vi "3kButtons2D22x22.vi"() -> ()   [LabVIEW 2011]
doc: "3000 buttons from haobo.li@pansino.com.cn\nhttp://www.linkedin.com/pub/haobo-li/17/8a/220\nthanks to\nhttp://www.fatcow.com/free-icons"
panel:
  out "zoom":bool
  out "youtube":bool
  out "yelp":bool
  out "yellow_submarine":bool
  out "yahoo_messenger":bool
  out "yacht":bool
  out "xing":bool
  out "xhtml_valid":bool
  out "xhtml_go":bool
  out "xhtml_delete":bool
  out "xhtml_add":bool
  out "xhtml":bool
  out "x_ray":bool
  out "www_page":bool
  out "wrench_orange":bool
  out "wrench":bool
  out "wrapping_tight":bool
  out "wrapping_square":bool
  out "wrapping_magazine":bool
  out "wrapping_inline":bool
  out "wrapping_in_front":bool
  out "wrapping_edit":bool
  out "wrapping_between":bool
  out "wrapping_behind":bool
  out "world_link":bool
  out "world_go":bool
  out "world_edit":bool
  out "world_delete":bool
  out "world_add":bool
  out "world":bool
  out "workspace":bool
  out "wordpress_blog":bool
  out "wordpress":bool
  out "wizard_women":bool
  out "wizard":bool
  out "wishlist_add":bool
  out "winrar_view":bool
  out "winrar_extract":bool
  out "winrar_add":bool
  out "wine_pairings":bool
  out "windy":bool
  out "widgets":bool
  out "widescreen":bool
  out "whistle":bool
  out "weight":bool
  out "weighing_mashine":bool
  out "webcam_error":bool
  out "webcam_delete":bool
  out "webcam_add":bool
  out "webcam":bool
  out "web_concierge":bool
  out "weather_sun":bool
  out "weather_snow":bool
  out "weather_rain":bool
  out "weather_lightning":bool
  out "weather_cloudy":bool
  out "weather_clouds":bool
  out "wand":bool
  out "wallet":bool
  out "walk":bool
  out "vslider":bool
  out "vrule":bool
  out "vlc":bool
  out "visa_electron":bool
  out "visa_2":bool
  out "visa":bool
  out "virus_protection":bool
  out "virb":bool
  out "vimeo":bool
  out "viewstack":bool
  out "videodisplay":bool
  out "video_mode":bool
  out "video":bool
  out "viddler":bool
  out "vhs":bool
  out "vector_delete":bool
  out "vector_add":bool
  out "vector":bool
  out "vdividedbox":bool
  out "vcard_edit":bool
  out "vcard_delete":bool
  out "vcard_add":bool
  out "vcard":bool
  out "vbox":bool
  out "user_zorro":bool
  out "user_yoda":bool
  out "user_wicket":bool
  out "user_waiter_female_black":bool
  out "user_waiter_female":bool
  out "user_waiter":bool
  out "user_viking_female":bool
  out "user_viking":bool
  out "user_vietnamese_female":bool
  out "user_vietnamese":bool
  out "user_trooper_captain":bool
  out "user_trooper":bool
  out "user_swimmer_female":bool
  out "user_swimmer_black":bool
  out "user_swimmer":bool
  out "user_superman":bool
  out "user_suit":bool
  out "user_student_female_black":bool
  out "user_student_female":bool
  out "user_student_black":bool
  out "user_student":bool
  out "user_striper_black":bool
  out "user_striper":bool
  out "user_stewardess_black":bool
  out "user_stewardess":bool
  out "user_squidward":bool
  out "user_sponge_bob":bool
  out "user_spiderman":bool
  out "user_soldier":bool
  out "user_silhouette":bool
  out "user_scream":bool
  out "user_samurai":bool
  out "user_sailor_black":bool
  out "user_sailor":bool
  out "user_robocop":bool
  out "user_redskin":bool
  out "user_red":bool
  out "user_rambo":bool
  out "user_racer":bool
  out "user_r2d2":bool
  out "user_queen_black":bool
  out "user_queen":bool
  out "user_pumpkin":bool
  out "user_priest_black":bool
  out "user_priest":bool
  out "user_policeman_black":bool
  out "user_policeman":bool
  out "user_police_female_black":bool
  out "user_police_female":bool
  out "user_police_england":bool
  out "user_plankton":bool
  out "user_pirate":bool
  out "user_pilot_civil":bool
  out "user_pilot":bool
  out "user_patrick":bool
  out "user_orange":bool
  out "user_oldwoman_black":bool
  out "user_oldwoman":bool
  out "user_oldman_black":bool
  out "user_oldman":bool
  out "user_officer_black":bool
  out "user_officer":bool
  out "user_nun_black":bool
  out "user_nun":bool
  out "user_nude_female_black":bool
  out "user_nude_female":bool
  out "user_nude_black":bool
  out "user_nude":bool
  out "user_ninja":bool
  out "user_muslim_female":bool
  out "user_muslim":bool
  out "user_mexican":bool
  out "user_medical_female_black":bool
  out "user_medical_female":bool
  out "user_medical_black":bool
  out "user_medical":bool
  out "user_maid":bool
  out "user_lisa":bool
  out "user_leprechaun":bool
  out "user_knight":bool
  out "user_king_black":bool
  out "user_king":bool
  out "user_judge_black":bool
  out "user_judge":bool
  out "user_jew":bool
  out "user_jester":bool
  out "user_jawa":bool
  out "user_jason":bool
  out "user_ironman":bool
  out "user_indian_female":bool
  out "user_indian":bool
  out "user_imprisoned_female_black":bool
  out "user_imprisoned_female":bool
  out "user_imprisoned_black":bool
  out "user_imprisoned":bool
  out "user_hendrix":bool
  out "user_halk":bool
  out "user_green":bool
  out "user_gray":bool
  out "user_goth":bool
  out "user_gomer":bool
  out "user_go":bool
  out "user_gladiator":bool
  out "user_geisha":bool
  out "user_freddy":bool
  out "user_firefighter_black":bool
  out "user_firefighter":bool
  out "user_female":bool
  out "user_eskimo_female":bool
  out "user_eskimo":bool
  out "user_emo":bool
  out "user_egyptian_female":bool
  out "user_egyptian":bool
  out "user_edit":bool
  out "user_dracula":bool
  out "user_diver":bool
  out "user_devil":bool
  out "user_detective_gray":bool
  out "user_detective":bool
  out "user_delete":bool
  out "user_death":bool
  out "user_darth_vader":bool
  out "user_crabs":bool
  out "user_cowboy_female":bool
  out "user_cowboy":bool
  out "user_cook_female_black":bool
  out "user_cook_female":bool
  out "user_cook_black":bool
  out "user_cook":bool
  out "user_comment":bool
  out "user_clown":bool
  out "user_chief_female_black":bool
  out "user_chief_female":bool
  out "user_chief_black":bool
  out "user_chief":bool
  out "user_catwomen":bool
  out "user_c3po":bool
  out "user_buddhist":bool
  out "user_boxer_black":bool
  out "user_boxer":bool
  out "user_blondy":bool
  out "user_bishop":bool
  out "user_bender":bool
  out "user_beach_lifeguard_female":bool
  out "user_beach_lifeguard":bool
  out "user_batman":bool
  out "user_bart":bool
  out "user_banker":bool
  out "user_ballplayer_black":bool
  out "user_ballplayer":bool
  out "user_astronaut":bool
  out "user_angel_female_black":bool
  out "user_angel_female":bool
  out "user_angel_black":bool
  out "user_angel":bool
  out "user_alien":bool
  out "user_add":bool
  out "user":bool
  out "usb_3":bool
  out "update":bool
  out "universal_binary":bool
  out "unicorn":bool
  out "understanding":bool
  out "underle_dictionary":bool
  out "umbrella":bool
  out "ufo":bool
  out "ubuntu":bool
  out "twitter_2":bool
  out "twitter_1":bool
  out "tux":bool
  out "turntable":bool
  out "tumblr":bool
  out "tubes":bool
  out "tub":bool
  out "trolley":bool
  out "trojan_horse":bool
  out "tree":bool
  out "travel":bool
  out "transmit_go":bool
  out "transmit_error":bool
  out "transmit_edit":bool
  out "transmit_delete":bool
  out "transmit_blue":bool
  out "transmit_add":bool
  out "transmit":bool
  out "transform_shear":bool
  out "transform_selection":bool
  out "transform_scale":bool
  out "transform_rotate_270":bool
  out "transform_rotate_180":bool
  out "transform_rotate_90":bool
  out "transform_rotate":bool
  out "transform_perspective":bool
  out "transform_path":bool
  out "transform_move":bool
  out "transform_layer":bool
  out "transform_flip":bool
  out "transform_crop_resize":bool
  out "transform_crop":bool
  out "traffic_usage":bool
  out "traffic_lights_yellow":bool
  out "traffic_lights_red":bool
  out "traffic_lights_green":bool
  out "traffic_lights":bool
  out "trade":bool
  out "tractor":bool
  out "toxic":bool
  out "tower":bool
  out "toucan":bool
  out "total_plan_cost":bool
  out "toster":bool
  out "tornado":bool
  out "torchere":bool
  out "tooth":bool
  out "toolbox":bool
  out "to_do_list_cheked_all":bool
  out "to_do_list_cheked_1":bool
  out "to_do_list":bool
  out "title_window":bool
  out "tire":bool
  out "tipper":bool
  out "timeline_marker":bool
  out "timeline":bool
  out "time_go":bool
  out "time_delete":bool
  out "time_add":bool
  out "time":bool
  out "tilelist":bool
  out "tick":bool
  out "thumb_up":bool
  out "thumb_down":bool
  out "three_tags":bool
  out "things_digital":bool
  out "things_beauty":bool
  out "theater":bool
  out "textfield_rename":bool
  out "textfield_key":bool
  out "textfield_delete":bool
  out "textfield_add":bool
  out "textfield":bool
  out "text_width":bool
  out "text_uppercase":bool
  out "text_underline":bool
  out "text_superscript":bool
  out "text_subscript":bool
  out "text_strikethroungh":bool
  out "text_smallcaps":bool
  out "text_signature":bool
  out "text_resize":bool
  out "text_replace":bool
  out "text_prose":bool
  out "text_pagination_100":bool
  out "text_pagination":bool
  out "text_padding_top":bool
  out "text_padding_right":bool
  out "text_padding_left":bool
  out "text_padding_bottom":bool
  out "text_lowercase":bool
  out "text_list_numbers":bool
  out "text_list_bullets":bool
  out "text_linespacing":bool
  out "text_letterspacing":bool
  out "text_letter_omega":bool
  out "text_large_cap":bool
  out "text_language":bool
  out "text_kerning":bool
  out "text_italic":bool
  out "text_indent_remove":bool
  out "text_indent":bool
  out "text_horizontalrule":bool
  out "text_heading_6":bool
  out "text_heading_5":bool
  out "text_heading_4":bool
  out "text_heading_3":bool
  out "text_heading_2":bool
  out "text_heading_1":bool
  out "text_dropcaps":bool
  out "text_drama":bool
  out "text_document_wrap":bool
  out "text_document":bool
  out "text_columns":bool
  out "text_bold":bool
  out "text_area":bool
  out "text_allcaps":bool
  out "text_align_right":bool
  out "text_align_left":bool
  out "text_align_justity":bool
  out "text_align_center":bool
  out "text":bool
  out "terminal_seats_red":bool
  out "terminal_seats_blue":bool
  out "terminal":bool
  out "temperature_5":bool
  out "temperature_4":bool
  out "temperature_3":bool
  out "temperature_2":bool
  out "temperature_1":bool
  out "television_delete":bool
  out "television_add":bool
  out "television":bool
  out "telephone_link":bool
  out "telephone_key":bool
  out "telephone_go":bool
  out "telephone_error":bool
  out "telephone_edit":bool
  out "telephone_delete":bool
  out "telephone_add":bool
  out "telephone":bool
  out "teddy_bear":bool
  out "technorati":bool
  out "teapot":bool
  out "tea_cup":bool
  out "tags_cloud":bool
  out "tag_yellow":bool
  out "tag_red":bool
  out "tag_purple":bool
  out "tag_pink":bool
  out "tag_orange":bool
  out "tag_green":bool
  out "tag_blue_edit":bool
  out "tag_blue_delete":bool
  out "tag_blue_add":bool
  out "tag_blue":bool
  out "tag":bool
  out "tabnavigator":bool
  out "tablets":bool
  out "table_torn":bool
  out "table_tab_search":bool
  out "table_tab_resize":bool
  out "table_tab":bool
  out "table_sum":bool
  out "table_split":bool
  out "table_sort":bool
  out "table_sheet":bool
  out "table_select_row":bool
  out "table_select_column":bool
  out "table_select_big":bool
  out "table_select_all":bool
  out "table_select":bool
  out "table_save":bool
  out "table_row_insert":bool
  out "table_row_delete":bool
  out "table_replace":bool
  out "table_relationship":bool
  out "table_refresh":bool
  out "table_paint_can":bool
  out "table_multiple":bool
  out "table_money":bool
  out "table_link":bool
  out "table_lightning":bool
  out "table_key":bool
  out "table_insert":bool
  out "table_import":bool
  out "table_heatmap":bool
  out "table_go":bool
  out "table_gear":bool
  out "table_export":bool
  out "table_excel":bool
  out "table_error":bool
  out "table_edit":bool
  out "table_delete":bool
  out "table_chart":bool
  out "table_add":bool
  out "table":bool
  out "tabbar":bool
  out "tab_go":bool
  out "tab_edit":bool
  out "tab_delete":bool
  out "tab_add":bool
  out "tab":bool
  out "system_time":bool
  out "system_monitor":bool
  out "sword":bool
  out "switch_220v":bool
  out "switch_120v":bool
  out "switch":bool
  out "swf_loader":bool
  out "support":bool
  out "sun_rain":bool
  out "sun_cloudy":bool
  out "sum":bool
  out "subwoofer":bool
  out "style_go":bool
  out "style_edit":bool
  out "style_delete":bool
  out "style_add":bool
  out "style":bool
  out "stumble_upon":bool
  out "street_stall":bool
  out "storage":bool
  out "stopwatch_start":bool
  out "stopwatch_pause":bool
  out "stopwatch_finish":bool
  out "stop":bool
  out "stethoscope_vintage":bool
  out "stethoscope":bool
  out "steering_wheel_3":bool
  out "steering_wheel_2":bool
  out "steering_wheel":bool
  out "steak_meat":bool
  out "steak_fish":bool
  out "status_online":bool
  out "status_offline":bool
  out "status_busy":bool
  out "status_away":bool
  out "statistics":bool
  out "star":bool
  out "stamp_pattern":bool
  out "ssl_certificates":bool
  out "sql_join_right_exclude":bool
  out "sql_join_right":bool
  out "sql_join_outer_exclude":bool
  out "sql_join_outer":bool
  out "sql_join_left_exclude":bool
  out "sql_join_left":bool
  out "sql_join_inner":bool
  out "sql_join":bool
  out "spring":bool
  out "sport_tennis":bool
  out "sport_soccer":bool
  out "sport_shuttlecock":bool
  out "sport_raquet":bool
  out "sport_golf":bool
  out "sport_football":bool
  out "sport_basketball":bool
  out "sport_8ball":bool
  out "sport":bool
  out "spill":bool
  out "spider_web":bool
  out "spellcheck_error":bool
  out "spellcheck":bool
  out "speedometer":bool
  out "speakers":bool
  out "spam_filter":bool
  out "spam":bool
  out "spacer":bool
  out "source_code":bool
  out "soup":bool
  out "sound_none":bool
  out "sound_mute":bool
  out "sound_low":bool
  out "sound_delete":bool
  out "sound_add":bool
  out "sound":bool
  out "sort_descending":bool
  out "sort_columns":bool
  out "sort_ascending":bool
  out "solar":bool
  out "soil_layers":bool
  out "soap":bool
  out "snowman":bool
  out "snow_rain":bool
  out "sneakers":bool
  out "snapshot":bool
  out "snake_and_cup":bool
  out "snail":bool
  out "small_tiles":bool
  out "small_car":bool
  out "small_business":bool
  out "slideshow":bool
  out "slackware":bool
  out "skype":bool
  out "skins":bool
  out "skate":bool
  out "size_vertical":bool
  out "size_horizontal":bool
  out "sitemap_color":bool
  out "sitemap":bool
  out "site_enhancer":bool
  out "site_backup_and_restore":bool
  out "siren":bool
  out "sign":bool
  out "shuriken":bool
  out "showel":bool
  out "shorts":bool
  out "shopping":bool
  out "shop_open":bool
  out "shop_closed":bool
  out "shirt_polo":bool
  out "shield_go":bool
  out "shield_delete":bool
  out "shield_add":bool
  out "shield":bool
  out "sheduled_task":bool
  out "sharpen":bool
  out "share":bool
  out "shape_ungroup":bool
  out "shape_square_link":bool
  out "shape_square_key":bool
  out "shape_square_go":bool
  out "shape_square_error":bool
  out "shape_square_edit":bool
  out "shape_square_delete":bool
  out "shape_square_add":bool
  out "shape_square":bool
  out "shape_rotate_clockwise":bool
  out "shape_rotate_anticlockwise":bool
  out "shape_move_front":bool
  out "shape_move_forwards":bool
  out "shape_move_backwards":bool
  out "shape_move_back":bool
  out "shape_handles":bool
  out "shape_group":bool
  out "shape_flip_vertical":bool
  out "shape_flip_horizontal":bool
  out "shape_align_top":bool
  out "shape_align_right":bool
  out "shape_align_middle":bool
  out "shape_align_left":bool
  out "shape_align_center":bool
  out "shape_align_bottom":bool
  out "shading":bool
  out "setting_tools":bool
  out "set_security_question":bool
  out "session_idle_time":bool
  out "server_uncompress":bool
  out "server_stanchion":bool
  out "server_link":bool
  out "server_lightning":bool
  out "server_key":bool
  out "server_information":bool
  out "server_go":bool
  out "server_error":bool
  out "server_edit":bool
  out "server_delete":bool
  out "server_database":bool
  out "server_connect":bool
  out "server_compress":bool
  out "server_components":bool
  out "server_chart":bool
  out "server_add":bool
  out "server":bool
  out "sertificate":bool
  out "select_restangular":bool
  out "select_lasso":bool
  out "select_invert":bool
  out "select_ellipse":bool
  out "select_continuous_area":bool
  out "select_by_intersection":bool
  out "select_by_difference":bool
  out "select_by_color":bool
  out "select_by_adding_to_selection":bool
  out "select":bool
  out "search_plus":bool
  out "search_minus":bool
  out "scull":bool
  out "scroller_bar":bool
  out "scripts":bool
  out "script_yellow":bool
  out "script_torn":bool
  out "script_save":bool
  out "script_red":bool
  out "script_palette":bool
  out "script_link":bool
  out "script_lightning":bool
  out "script_key":bool
  out "script_green":bool
  out "script_go":bool
  out "script_gear":bool
  out "script_error":bool
  out "script_edit":bool
  out "script_delete":bool
  out "script_code_red":bool
  out "script_code":bool
  out "script_black":bool
  out "script_add":bool
  out "script":bool
  out "screwdriver":bool
  out "screen_error":bool
  out "scanner":bool
  out "scalpel":bool
  out "scale_image":bool
  out "save_money":bool
  out "save_as":bool
  out "satellite_dish":bool
  out "satellite":bool
  out "santa":bool
  out "salver":bool
  out "sallary_deferrais":bool
  out "safe":bool
  out "safari_browser":bool
  out "ruby_put":bool
  out "ruby_link":bool
  out "ruby_key":bool
  out "ruby_go":bool
  out "ruby_get":bool
  out "ruby_gear":bool
  out "ruby_delete":bool
  out "ruby_add":bool
  out "ruby":bool
  out "rubber_duck":bool
  out "rss_valid":bool
  out "rss_go":bool
  out "rss_delete":bool
  out "rss_add":bool
  out "rss":bool
  out "routing_turning_right":bool
  out "routing_turning_left":bool
  out "routing_turnaround_right":bool
  out "routing_turnaround_left":bool
  out "routing_turn_u":bool
  out "routing_turn_right_2":bool
  out "routing_turn_right":bool
  out "routing_turn_left_crossroads":bool
  out "routing_turn_left_2":bool
  out "routing_turn_left":bool
  out "routing_turn_arround_right":bool
  out "routing_turn_arround_left":bool
  out "routing_intersection_right":bool
  out "routing_go_straight_right":bool
  out "routing_go_straight_left":bool
  out "routing_go_right":bool
  out "routing_go_left":bool
  out "routing_forward":bool
  out "routing_around":bool
  out "router":bool
  out "rotate_90":bool
  out "rosette":bool
  out "role":bool
  out "rocking_chair":bool
  out "robo_to":bool
  out "roadworks":bool
  out "road_sign":bool
  out "rip":bool
  out "ring":bool
  out "richtext_editor":bool
  out "ribbon":bool
  out "resultset_previous":bool
  out "resultset_next":bool
  out "resultset_last":bool
  out "resultset_first":bool
  out "restaurant_menu":bool
  out "resources":bool
  out "resource_usage":bool
  out "resize_picture":bool
  out "reseller_programm":bool
  out "reseller_account_template":bool
  out "reseller_account":bool
  out "report_word":bool
  out "report_user":bool
  out "report_torn":bool
  out "report_picture":bool
  out "report_magnify":bool
  out "report_link":bool
  out "report_key":bool
  out "report_go":bool
  out "report_edit":bool
  out "report_disk":bool
  out "report_delete":bool
  out "report_add":bool
  out "report":bool
  out "remote":bool
  out "reddit":bool
  out "red_line":bool
  out "recycle_bag":bool
  out "recycle":bool
  out "real_estate":bool
  out "readernaut":bool
  out "rainbow_cloud":bool
  out "rainbow":bool
  out "rain":bool
  out "radiolocator":bool
  out "radiobutton_group":bool
  out "radiobutton":bool
  out "radioactivity":bool
  out "radio_2":bool
  out "radio_1":bool
  out "rabbit":bool
  out "question":bool
  out "qip_online":bool
  out "qip_offline":bool
  out "qip_occupied":bool
  out "qip_not_available":bool
  out "qip_invisible_for_all":bool
  out "qip_invisible":bool
  out "qip_free_for_chat":bool
  out "qip_eating":bool
  out "qip_dnd":bool
  out "qip_bad_mood":bool
  out "qip_away":bool
  out "qip_at_work":bool
  out "qip_at_home":bool
  out "qip_angry":bool
  out "qik":bool
  out "purse":bool
  out "progressbar":bool
  out "profiles":bool
  out "production_copyleft":bool
  out "processor":bool
  out "private":bool
  out "printer_error":bool
  out "printer_empty":bool
  out "printer_delete":bool
  out "printer_add":bool
  out "printer":bool
  out "print_size":bool
  out "price_watch":bool
  out "price_comparison":bool
  out "price_alert":bool
  out "premium_support":bool
  out "preferences":bool
  out "power_surge":bool
  out "posterous":bool
  out "postage_stamp":bool
  out "port":bool
  out "popcorn":bool
  out "pop_mail":bool
  out "poo":bool
  out "poker":bool
  out "plurk":bool
  out "plugin_link":bool
  out "plugin_go":bool
  out "plugin_error":bool
  out "plugin_edit":bool
  out "plugin_disabled":bool
  out "plugin_delete":bool
  out "plugin_add":bool
  out "plugin":bool
  out "plotchart":bool
  out "playstation":bool
  out "Plant":bool
  out "plane":bool
  out "places":bool
  out "pizza":bool
  out "pirate_flag":bool
  out "pint":bool
  out "pill_go":bool
  out "pill_delete":bool
  out "pill_add":bool
  out "pill":bool
  out "pilcrow":bool
  out "piechart":bool
  out "piece_of_cake":bool
  out "pictures":bool
  out "picture_save":bool
  out "picture_link":bool
  out "picture_key":bool
  out "picture_go":bool
  out "picture_frame":bool
  out "picture_error":bool
  out "picture_empty":bool
  out "picture_edit":bool
  out "picture_delete":bool
  out "picture_add":bool
  out "picture":bool
  out "picasa":bool
  out "piano":bool
  out "pi_math":bool
  out "photos":bool
  out "photo_link":bool
  out "photo_delete":bool
  out "photo_add":bool
  out "photo":bool
  out "phone_vintage":bool
  out "phone_sound":bool
  out "phone_delete":bool
  out "phone_Android":bool
  out "phone_add":bool
  out "phone":bool
  out "personals":bool
  out "personal_finance":bool
  out "perfomance":bool
  out "pepper":bool
  out "pencil_go":bool
  out "pencil_delete":bool
  out "pencil_add":bool
  out "pencil":bool
  out "pearl":bool
  out "peak_cap":bool
  out "peacock":bool
  out "pci":bool
  out "pc_linux_os":bool
  out "paypal-2":bool
  out "paypal":bool
  out "paste_word":bool
  out "paste_plain":bool
  out "participation_rate":bool
  out "parrot":bool
  out "paper_airplane":bool
  out "panel":bool
  out "pandora":bool
  out "palette":bool
  out "paintcan":bool
  out "paintbrush":bool
  out "page_world":bool
  out "page_word":bool
  out "page_white_zip":bool
  out "page_white_wrench":bool
  out "page_white_world":bool
  out "page_white_word":bool
  out "page_white_width":bool
  out "page_white_visualstudio":bool
  out "page_white_vector":bool
  out "page_white_tux":bool
  out "page_white_text_width":bool
  out "page_white_text":bool
  out "page_white_star":bool
  out "page_white_stack":bool
  out "page_white_ruby":bool
  out "page_white_put":bool
  out "page_white_powerpoint":bool
  out "page_white_picture":bool
  out "page_white_php":bool
  out "page_white_paste":bool
  out "page_white_paintbrush":bool
  out "page_white_paint":bool
  out "page_white_office":bool
  out "page_white_medal":bool
  out "page_white_magnify":bool
  out "page_white_link":bool
  out "page_white_lightning":bool
  out "page_white_key":bool
  out "page_white_horizontal":bool
  out "page_white_h":bool
  out "page_white_go":bool
  out "page_white_get":bool
  out "page_white_gear":bool
  out "page_white_flash":bool
  out "page_white_find":bool
  out "page_white_excel":bool
  out "page_white_error":bool
  out "page_white_edit":bool
  out "page_white_dvd":bool
  out "page_white_delete":bool
  out "page_white_database":bool
  out "page_white_cup":bool
  out "page_white_csharp":bool
  out "page_white_cplusplus":bool
  out "page_white_copy":bool
  out "page_white_compress":bool
  out "page_white_code_red":bool
  out "page_white_code":bool
  out "page_white_cd":bool
  out "page_white_camera":bool
  out "page_white_c":bool
  out "page_white_add":bool
  out "page_white_actionscript":bool
  out "page_white_acrobat":bool
  out "page_white":bool
  out "page_save":bool
  out "page_refresh":bool
  out "page_red":bool
  out "page_paste":bool
  out "page_paintbrush":bool
  out "page_magnifier":bool
  out "page_link":bool
  out "page_lightning":bool
  out "page_key":bool
  out "page_green":bool
  out "page_go":bool
  out "page_gear":bool
  out "page_find":bool
  out "page_excel":bool
  out "page_error":bool
  out "page_edit":bool
  out "page_delete":bool
  out "page_copy":bool
  out "page_code":bool
  out "page_attach":bool
  out "page_add":bool
  out "page":bool
  out "package_link":bool
  out "package_green":bool
  out "package_go":bool
  out "package_delete":bool
  out "package_add":bool
  out "package":bool
  out "other_phone":bool
  out "orthodox_church":bool
  out "ornament_gold":bool
  out "orkut":bool
  out "origami":bool
  out "orbit":bool
  out "opera":bool
  out "openid":bool
  out "open_suse":bool
  out "open_folder":bool
  out "omelet":bool
  out "oil":bool
  out "numeric_stepper":bool
  out "note_torn":bool
  out "note_go":bool
  out "note_error":bool
  out "note_edit":bool
  out "note_delete":bool
  out "note_add":bool
  out "note":bool
  out "non_derivative":bool
  out "nokia_s60":bool
  out "node-tree":bool
  out "no_smoking":bool
  out "no_requirements":bool
  out "no_image":bool
  out "no_drm_trm":bool
  out "no_commercial":bool
  out "newsvine":bool
  out "newspaper_link":bool
  out "newspaper_go":bool
  out "newspaper_delete":bool
  out "newspaper_add":bool
  out "newspaper":bool
  out "new":bool
  out "network-share":bool
  out "networking_red":bool
  out "networking_green":bool
  out "networking":bool
  out "network_wireless":bool
  out "network_ip":bool
  out "network_hub":bool
  out "network_folder":bool
  out "network_firewall":bool
  out "network_ethernet":bool
  out "network_clouds":bool
  out "network_cloud":bool
  out "network_adapter":bool
  out "netvibes":bool
  out "nameboard_open":bool
  out "myspace":bool
  out "my_name_is_e":bool
  out "mustache":bool
  out "music":bool
  out "multitool":bool
  out "multiplied_by_100":bool
  out "multiplied_by_10":bool
  out "multiplied_by_5":bool
  out "multiplied_by_3":bool
  out "multiplied_by_2":bool
  out "msn_messenger":bool
  out "ms_frontpage":bool
  out "ms_exchange":bool
  out "movies":bool
  out "move_to_folder":bool
  out "mouse_select_scroll":bool
  out "mouse_select_right":bool
  out "mouse_select_left":bool
  out "mouse_error":bool
  out "mouse_delete":bool
  out "mouse_add":bool
  out "mouse_2":bool
  out "mouse":bool
  out "motherboard":bool
  out "mosque":bool
  out "moon":bool
  out "monitor_window_3d":bool
  out "monitor_window":bool
  out "monitor_wallpaper":bool
  out "monitor_sidebar":bool
  out "monitor_screensaver":bool
  out "monitor_link":bool
  out "monitor_lightning":bool
  out "monitor_go":bool
  out "monitor_error":bool
  out "monitor_edit":bool
  out "monitor_delete":bool
  out "monitor_add":bool
  out "monitor":bool
  out "moneybox":bool
  out "money_yen":bool
  out "money_pound":bool
  out "money_in_envelope":bool
  out "money_euro":bool
  out "money_dollar":bool
  out "money_delete":bool
  out "money_bookers":bool
  out "money_bag":bool
  out "money_add":bool
  out "money":bool
  out "molecule":bool
  out "mobile_me":bool
  out "mixx":bool
  out "mixture":bool
  out "mixer":bool
  out "milestone":bool
  out "microwave":bool
  out "microscope":bool
  out "microphone":bool
  out "microformats":bool
  out "micro_sd_blue":bool
  out "micro_sd":bool
  out "metronome":bool
  out "metro":bool
  out "messenger":bool
  out "menubar":bool
  out "menu_item":bool
  out "menu":bool
  out "medical_record":bool
  out "medal_silver_delete":bool
  out "medal_silver_add":bool
  out "medal_silver_3":bool
  out "medal_silver_2":bool
  out "medal_silver_1":bool
  out "medal_gold_delete":bool
  out "medal_gold_add":bool
  out "medal_gold_3":bool
  out "medal_gold_2":bool
  out "medal_gold_1":bool
  out "medal_bronze_delete":bool
  out "medal_bronze_add":bool
  out "medal_bronze_3":bool
  out "medal_bronze_2":bool
  out "medal_bronze_1":bool
  out "medal_award_silver":bool
  out "medal_award_gold":bool
  out "medal_award_bronze":bool
  out "measure_crop":bool
  out "measure":bool
  out "master_card":bool
  out "mask":bool
  out "marketwatch":bool
  out "mario":bool
  out "map_torn":bool
  out "map_magnify":bool
  out "map_go":bool
  out "map_edit":bool
  out "map_delete":bool
  out "map_add":bool
  out "map":bool
  out "mandriva":bool
  out "male":bool
  out "mail-trash":bool
  out "mail_yellow":bool
  out "mail_torn":bool
  out "mail_server_setting":bool
  out "mail_red":bool
  out "mail_green":bool
  out "mail_box":bool
  out "mail_black":bool
  out "magnifier_zoom_out":bool
  out "magnifier_zoom_in":bool
  out "magnifier":bool
  out "magnet":bool
  out "magic_wand_2":bool
  out "luggage_brown_tag":bool
  out "luggage_brown":bool
  out "luggage":bool
  out "lorry_link":bool
  out "lorry_go":bool
  out "lorry_flatbed":bool
  out "lorry_error":bool
  out "lorry_delete":bool
  out "lorry_add":bool
  out "lorry":bool
  out "lollypop":bool
  out "lollipop":bool
  out "lock_open":bool
  out "lock_go":bool
  out "lock_edit":bool
  out "lock_delete":bool
  out "lock_break":bool
  out "lock_add":bool
  out "lock":bool
  out "location_pin":bool
  out "locate":bool
  out "livejournal":bool
  out "list":bool
  out "linux_mint":bool
  out "linkedin":bool
  out "linkbar":bool
  out "link_unchain":bool
  out "link_juice":bool
  out "link_go":bool
  out "link_edit":bool
  out "link_delete":bool
  out "link_button":bool
  out "link_break":bool
  out "link_add":bool
  out "link":bool
  out "linechart":bool
  out "line_split":bool
  out "lightning_go":bool
  out "lightning_delete":bool
  out "lightning_add":bool
  out "lightning":bool
  out "lighthouse_shine":bool
  out "lighthouse":bool
  out "lightbulb_off":bool
  out "lightbulb_delete":bool
  out "lightbulb_add":bool
  out "lightbulb":bool
  out "light_circle_green":bool
  out "life_vest":bool
  out "license_management":bool
  out "license_key":bool
  out "legend":bool
  out "led":bool
  out "layouts_split_vertical":bool
  out "layouts_split":bool
  out "layouts_select_sidebar":bool
  out "layouts_select_footer":bool
  out "layouts_select_content":bool
  out "layouts_select":bool
  out "layouts_join_vertical":bool
  out "layouts_join":bool
  out "layouts_hf_3":bool
  out "layouts_hf_2_equal":bool
  out "layouts_header_footer_3":bool
  out "layouts_header_footer_2":bool
  out "layouts_header_footer":bool
  out "layouts_header_3_mix":bool
  out "layouts_header_3":bool
  out "layouts_header_2_equal":bool
  out "layouts_header_2":bool
  out "layouts_header":bool
  out "layouts_design":bool
  out "layouts_6":bool
  out "layouts_4":bool
  out "layouts_3_mix":bool
  out "layouts_3":bool
  out "layouts_2":bool
  out "layouts":bool
  out "layout_sidebar":bool
  out "layout_link":bool
  out "layout_header":bool
  out "layout_error":bool
  out "layout_edit":bool
  out "layout_delete":bool
  out "layout_content":bool
  out "layout_add":bool
  out "layout":bool
  out "layers_map":bool
  out "layers":bool
  out "layer_wms":bool
  out "layer_vector":bool
  out "layer_transparent":bool
  out "layer_to_image_size":bool
  out "layer_stack_arrange_back":bool
  out "layer_stack_arrange":bool
  out "layer_shred":bool
  out "layer_shape_text":bool
  out "layer_shape_round":bool
  out "layer_shape_polyline":bool
  out "layer_shape_ellipse":bool
  out "layer_shape":bool
  out "layer_shaded_relief":bool
  out "layer_shade":bool
  out "layer_select":bool
  out "layer_save":bool
  out "layer_rgb":bool
  out "layer_resize_replicate_v":bool
  out "layer_resize_replicate_h":bool
  out "layer_resize_actual":bool
  out "layer_resize":bool
  out "layer_remove":bool
  out "layer_redraw":bool
  out "layer_raster_3d":bool
  out "layer_raster":bool
  out "layer_open":bool
  out "layer_mask":bool
  out "layer_label":bool
  out "layer_import":bool
  out "layer_histogram":bool
  out "layer_his":bool
  out "layer_group":bool
  out "layer_grid":bool
  out "layer_gps":bool
  out "layer_export":bool
  out "layer_edit":bool
  out "layer_delete":bool
  out "layer_database":bool
  out "layer_create":bool
  out "layer_command":bool
  out "layer_chart":bool
  out "layer_cell_cats":bool
  out "layer_aspect_arrow":bool
  out "layer_arrange_back":bool
  out "layer_arrange":bool
  out "layer_add":bool
  out "layer":bool
  out "last_fm":bool
  out "large_tiles":bool
  out "laptop":bool
  out "language":bool
  out "landmarks":bool
  out "ladybird":bool
  out "knot":bool
  out "kids":bool
  out "keyboard_magnify":bool
  out "keyboard_delete":bool
  out "keyboard_add":bool
  out "keyboard":bool
  out "key_z":bool
  out "key_y":bool
  out "key_x":bool
  out "key_w":bool
  out "key_v":bool
  out "key_u":bool
  out "key_t":bool
  out "key_solid":bool
  out "key_s":bool
  out "key_r":bool
  out "key_q":bool
  out "key_p":bool
  out "key_o":bool
  out "key_n":bool
  out "key_m":bool
  out "key_l":bool
  out "key_k":bool
  out "key_j":bool
  out "key_i":bool
  out "key_h":bool
  out "key_go":bool
  out "key_g":bool
  out "key_f":bool
  out "key_escape":bool
  out "key_e":bool
  out "key_delete":bool
  out "key_d":bool
  out "key_c":bool
  out "key_b":bool
  out "key_add":bool
  out "key_a":bool
  out "key":bool
  out "json":bool
  out "joystick_error":bool
  out "joystick_delete":bool
  out "joystick_add":bool
  out "joystick":bool
  out "jeans":bool
  out "jason_mask":bool
  out "jar_open":bool
  out "jar_empty":bool
  out "jacket":bool
  out "italy":bool
  out "ipod_sound":bool
  out "ipod_cast_delete":bool
  out "ipod_cast_add":bool
  out "ipod_cast":bool
  out "ipod":bool
  out "iphone":bool
  out "ipad":bool
  out "ip_class":bool
  out "ip_block":bool
  out "ip":bool
  out "investment_menu_quality":bool
  out "internet_explorer":bool
  out "interface_preferences":bool
  out "installer_box":bool
  out "insert_object":bool
  out "insert_element":bool
  out "injection":bool
  out "information":bool
  out "info_rhombus":bool
  out "index-cards":bool
  out "inbox_upload":bool
  out "inbox_table":bool
  out "inbox_slide":bool
  out "inbox_images":bool
  out "inbox_film":bool
  out "inbox_empty":bool
  out "inbox_download":bool
  out "inbox_document_text":bool
  out "inbox_document_music":bool
  out "inbox_document":bool
  out "images_flickr":bool
  out "images":bool
  out "image_link":bool
  out "image_edit":bool
  out "image_delete":bool
  out "image_add":bool
  out "image":bool
  out "im_messenger":bool
  out "ilike":bool
  out "icecream":bool
  out "ice_cube":bool
  out "hummingbird":bool
  out "http_status_unavailable":bool
  out "http_status_temporary":bool
  out "http_status_server_error":bool
  out "http_status_permanent":bool
  out "http_status_ok_success":bool
  out "http_status_not_found":bool
  out "html_valid":bool
  out "html_go":bool
  out "html_delete":bool
  out "html_add":bool
  out "html_5":bool
  out "html":bool
  out "hslider":bool
  out "hrule":bool
  out "house_two":bool
  out "house_one":bool
  out "house_link":bool
  out "house_go":bool
  out "house":bool
  out "hourglass_link":bool
  out "hourglass_go":bool
  out "hourglass_delete":bool
  out "hourglass_add":bool
  out "hourglass":bool
  out "hotjobs":bool
  out "hot":bool
  out "hostname":bool
  out "hospital":bool
  out "horoscopes":bool
  out "horn":bool
  out "horizontal_list":bool
  out "home_page":bool
  out "holly":bool
  out "hlocchart":bool
  out "hippocampus":bool
  out "highlighter_text":bool
  out "highlighter":bool
  out "help":bool
  out "helmet_mine":bool
  out "helmet":bool
  out "helicopter":bool
  out "heart_half":bool
  out "heart_empty":bool
  out "heart_delete":bool
  out "heart_break":bool
  out "heart_add":bool
  out "heart":bool
  out "health":bool
  out "headphone_mic":bool
  out "headphone":bool
  out "hdividedbox":bool
  out "hd_ready":bool
  out "hd_1080":bool
  out "hd_720":bool
  out "hbox":bool
  out "hat":bool
  out "hardware_building_oem":bool
  out "handbag":bool
  out "hand_property":bool
  out "hand_point_270":bool
  out "hand_point_180":bool
  out "hand_point_090":bool
  out "hand_point":bool
  out "hand_ily":bool
  out "hand_fuck":bool
  out "hand":bool
  out "hammer":bool
  out "hamburger":bool
  out "half_moon":bool
  out "gun":bool
  out "group_link":bool
  out "group_key":bool
  out "group_go":bool
  out "group_gear":bool
  out "group_error":bool
  out "group_edit":bool
  out "group_delete":bool
  out "group_add":bool
  out "group":bool
  out "grooveshark":bool
  out "grid":bool
  out "grenade":bool
  out "green_yellow":bool
  out "green_wormhole":bool
  out "green":bool
  out "grass":bool
  out "gps_handheld":bool
  out "gps_automotive":bool
  out "gowalla":bool
  out "google_webmaster_tools":bool
  out "google_web_elements":bool
  out "google_wave":bool
  out "google_voice":bool
  out "google_talk":bool
  out "google_plus":bool
  out "google_new":bool
  out "google_map_satellite":bool
  out "google_map":bool
  out "google_custom_search":bool
  out "google_adsense":bool
  out "google":bool
  out "globe_place":bool
  out "globe_network":bool
  out "globe_model":bool
  out "global_telecom":bool
  out "glass_narrow":bool
  out "gift_add":bool
  out "geotag":bool
  out "georectify":bool
  out "gentoo_linux":bool
  out "gear_in":bool
  out "gcp_rms":bool
  out "gcp":bool
  out "gas":bool
  out "gamespot":bool
  out "game_monitor":bool
  out "ftp":bool
  out "fruit_lime":bool
  out "fruit_grape":bool
  out "friendfeed":bool
  out "freebsd":bool
  out "forrst":bool
  out "formheading":bool
  out "form":bool
  out "forklift":bool
  out "font_superscript":bool
  out "font_subscript":bool
  out "font_red_delete":bool
  out "font_red":bool
  out "font_go":bool
  out "font_delete":bool
  out "font_colors":bool
  out "font_add":bool
  out "font":bool
  out "folding_fan":bool
  out "folders_explorer":bool
  out "folders":bool
  out "folder_wrench":bool
  out "folder_vertical_zipper":bool
  out "folder_vertical_torn":bool
  out "folder_vertical_rename":bool
  out "folder_vertical_open":bool
  out "folder_vertical_document":bool
  out "folder_user":bool
  out "folder_torn":bool
  out "folder_table":bool
  out "folder_star":bool
  out "folder_stand":bool
  out "folder_search":bool
  out "folder_red":bool
  out "folder_picture":bool
  out "folder_palette":bool
  out "folder_page_white":bool
  out "folder_page":bool
  out "folder_link":bool
  out "folder_lightbulb":bool
  out "folder_key":bool
  out "folder_image":bool
  out "folder_heart":bool
  out "folder_green":bool
  out "folder_go":bool
  out "folder_find":bool
  out "folder_feed":bool
  out "folder_explore":bool
  out "folder_error":bool
  out "folder_edit":bool
  out "folder_delete":bool
  out "folder_database":bool
  out "folder_camera":bool
  out "folder_bug":bool
  out "folder_brick":bool
  out "folder_blue":bool
  out "folder_black":bool
  out "folder_bell":bool
  out "folder_add":bool
  out "folder":bool
  out "fog":bool
  out "flower":bool
  out "flood_it":bool
  out "flickr":bool
  out "flex_builder":bool
  out "flex":bool
  out "flask_empty":bool
  out "flask":bool
  out "flashlight_shine":bool
  out "flashlight":bool
  out "flashdisk":bool
  out "flamingo":bool
  out "flag_zimbabwe":bool
  out "flag_zambia":bool
  out "flag_yemen":bool
  out "flag_yellow":bool
  out "flag_wwf":bool
  out "flag_wto":bool
  out "flag_wallis_and_futuna":bool
  out "flag_wales":bool
  out "flag_virgin_islands":bool
  out "flag_vietnam":bool
  out "flag_venezuela":bool
  out "flag_vatican_city":bool
  out "flag_vanuatu":bool
  out "flag_uzbekistan":bool
  out "flag_usa":bool
  out "flag_uruquay":bool
  out "flag_united_nations":bool
  out "flag_united_arab_emirates":bool
  out "flag_unesco":bool
  out "flag_ukraine":bool
  out "flag_uganda":bool
  out "flag_tuvalu":bool
  out "flag_turks_and_caicos_islands":bool
  out "flag_turkmenistan":bool
  out "flag_turkey":bool
  out "flag_tunisia":bool
  out "flag_trinidad_and_tobago":bool
  out "flag_tonga":bool
  out "flag_togo":bool
  out "flag_tibet":bool
  out "flag_thailand":bool
  out "flag_tanzania":bool
  out "flag_tajikistan":bool
  out "flag_taiwan":bool
  out "flag_syria":bool
  out "flag_switzerland":bool
  out "flag_sweden":bool
  out "flag_swaziland":bool
  out "flag_suriname":bool
  out "flag_sudan":bool
  out "flag_sri_lanka":bool
  out "flag_spain":bool
  out "flag_south_korea":bool
  out "flag_south_georgia":bool
  out "flag_south_africa":bool
  out "flag_somalia":bool
  out "flag_solomon_islands":bool
  out "flag_slovenia":bool
  out "flag_slovakia":bool
  out "flag_singapore":bool
  out "flag_sierra_leone":bool
  out "flag_seychelles":bool
  out "flag_serbia_montenegro":bool
  out "flag_senegal":bool
  out "flag_scotland":bool
  out "flag_saudi_arabia":bool
  out "flag_sao_tome_and_principe":bool
  out "flag_san_marino":bool
  out "flag_samoa":bool
  out "flag_saint_vincent_and_grenadines":bool
  out "flag_saint_pierre_and_miquelon":bool
  out "flag_saint_lucia":bool
  out "flag_saint_kitts_and_nevis":bool
  out "flag_saint_helena":bool
  out "flag_rwanda":bool
  out "flag_russia":bool
  out "flag_romania":bool
  out "flag_red_cross":bool
  out "flag_red":bool
  out "flag_qatar":bool
  out "flag_purple":bool
  out "flag_puerto_rico":bool
  out "flag_portugal":bool
  out "flag_poland":bool
  out "flag_pitcairn_islands":bool
  out "flag_pink":bool
  out "flag_philippines":bool
  out "flag_peru":bool
  out "flag_paraquay":bool
  out "flag_papua_new_guinea":bool
  out "flag_panama":bool
  out "flag_palau":bool
  out "flag_pakistan":bool
  out "flag_orange":bool
  out "flag_oman":bool
  out "flag_olympic":bool
  out "flag_norway":bool
  out "flag_northern_mariana_islands":bool
  out "flag_north_korea":bool
  out "flag_norfolk_islands":bool
  out "flag_niue":bool
  out "flag_nigeria":bool
  out "flag_niger":bool
  out "flag_nicaragua":bool
  out "flag_new_zealand":bool
  out "flag_new":bool
  out "flag_netherlands_antilles":bool
  out "flag_netherlands":bool
  out "flag_nepal":bool
  out "flag_nauru":bool
  out "flag_nato":bool
  out "flag_namibia":bool
  out "flag_mozambique":bool
  out "flag_morocco":bool
  out "flag_montserrat":bool
  out "flag_mongolia":bool
  out "flag_monaco":bool
  out "flag_moldova":bool
  out "flag_micronesia":bool
  out "flag_mexico":bool
  out "flag_mauritius":bool
  out "flag_mauretania":bool
  out "flag_martinique":bool
  out "flag_marshall_islands":bool
  out "flag_malta":bool
  out "flag_mali":bool
  out "flag_maledives":bool
  out "flag_malaysia":bool
  out "flag_malawi":bool
  out "flag_madagascar":bool
  out "flag_macedonia":bool
  out "flag_macau":bool
  out "flag_luxembourg":bool
  out "flag_lithuania":bool
  out "flag_liechtenstein":bool
  out "flag_libya":bool
  out "flag_liberia":bool
  out "flag_lesotho":bool
  out "flag_lebanon":bool
  out "flag_latvia":bool
  out "flag_laos":bool
  out "flag_kyrgyzstan":bool
  out "flag_kuwait":bool
  out "flag_kiribati":bool
  out "flag_kenya":bool
  out "flag_kazakhstan":bool
  out "flag_jordan":bool
  out "flag_jersey":bool
  out "flag_japan":bool
  out "flag_jamaica":bool
  out "flag_italy":bool
  out "flag_israel":bool
  out "flag_isle_of_man":bool
  out "flag_ireland":bool
  out "flag_iraq":bool
  out "flag_iran":bool
  out "flag_indonesia":bool
  out "flag_india":bool
  out "flag_iceland":bool
  out "flag_hungary":bool
  out "flag_hot":bool
  out "flag_hong_kong":bool
  out "flag_honduras":bool
  out "flag_haiti":bool
  out "flag_guyana":bool
  out "flag_guinea_bissau":bool
  out "flag_guinea":bool
  out "flag_guernsey":bool
  out "flag_guatemala":bool
  out "flag_guam":bool
  out "flag_grenada":bool
  out "flag_greenland":bool
  out "flag_green":bool
  out "flag_greece":bool
  out "flag_great_britain":bool
  out "flag_gibraltar":bool
  out "flag_ghana":bool
  out "flag_germany":bool
  out "flag_georgia":bool
  out "flag_gambia":bool
  out "flag_gabon":bool
  out "flag_french_polynesia":bool
  out "flag_france":bool
  out "flag_finland":bool
  out "flag_finish":bool
  out "flag_fiji":bool
  out "flag_faroe_islands":bool
  out "flag_falkland_islands":bool
  out "flag_european_union":bool
  out "flag_ethiopia":bool
  out "flag_estonia":bool
  out "flag_eritrea":bool
  out "flag_equatorial_guinea":bool
  out "flag_equador":bool
  out "flag_england":bool
  out "flag_el_salvador":bool
  out "flag_egypt":bool
  out "flag_east_timor":bool
  out "flag_dominican_republic":bool
  out "flag_dominica":bool
  out "flag_djibouti":bool
  out "flag_denmark":bool
  out "flag_czech_republic":bool
  out "flag_cyprus":bool
  out "flag_cuba":bool
  out "flag_croatia":bool
  out "flag_cote_divoire":bool
  out "flag_costa_rica":bool
  out "flag_cope_verde":bool
  out "flag_cook_islands":bool
  out "flag_congo_republic":bool
  out "flag_congo_democratic_republic":bool
  out "flag_comoros":bool
  out "flag_colombia":bool
  out "flag_china":bool
  out "flag_chile":bool
  out "flag_chad":bool
  out "flag_central_african_republic":bool
  out "flag_cayman_islands":bool
  out "flag_canada":bool
  out "flag_cameroon":bool
  out "flag_cambodia":bool
  out "flag_burundi":bool
  out "flag_burma":bool
  out "flag_burkina_faso":bool
  out "flag_bulgaria":bool
  out "flag_brunei":bool
  out "flag_british_virgin_islands":bool
  out "flag_british_indian_ocean":bool
  out "flag_brazil":bool
  out "flag_boy_scout":bool
  out "flag_botswana":bool
  out "flag_bosnia":bool
  out "flag_bolivia":bool
  out "flag_blue":bool
  out "flag_bhutan":bool
  out "flag_bermuda":bool
  out "flag_benin":bool
  out "flag_belize":bool
  out "flag_belgium":bool
  out "flag_belarus":bool
  out "flag_barbados":bool
  out "flag_bangladesh":bool
  out "flag_bahrain":bool
  out "flag_bahamas":bool
  out "flag_azerbaijan":bool
  out "flag_austria":bool
  out "flag_australia":bool
  out "flag_aruba":bool
  out "flag_armenia":bool
  out "flag_argentina":bool
  out "flag_antigua_and_barbuda":bool
  out "flag_anguilla":bool
  out "flag_angola":bool
  out "flag_andorra":bool
  out "flag_american_samoa":bool
  out "flag_algeria":bool
  out "flag_albania":bool
  out "flag_airfield_vehicle_safety":bool
  out "flag_afghanistan":bool
  out "flag_3":bool
  out "flag_2":bool
  out "flag_1":bool
  out "fishfinder":bool
  out "firewall_burn":bool
  out "firewall":bool
  out "firefox":bool
  out "fire_extinguisher":bool
  out "fire_damage":bool
  out "fire":bool
  out "fingerprint":bool
  out "find":bool
  out "finance":bool
  out "filter_delete":bool
  out "filter_add":bool
  out "filter":bool
  out "film_save":bool
  out "film_photo":bool
  out "film_link":bool
  out "film_key":bool
  out "film_go":bool
  out "film_error":bool
  out "film_edit":bool
  out "film_delete":bool
  out "film_add":bool
  out "film":bool
  out "fill":bool
  out "file_manager":bool
  out "file_extension_zip":bool
  out "file_extension_xpi":bool
  out "file_extension_xls":bool
  out "file_extension_wps":bool
  out "file_extension_wmv":bool
  out "file_extension_wma":bool
  out "file_extension_wav":bool
  out "file_extension_vob":bool
  out "file_extension_vcd":bool
  out "file_extension_txt":bool
  out "file_extension_ttf":bool
  out "file_extension_torrent":bool
  out "file_extension_tmp":bool
  out "file_extension_tif":bool
  out "file_extension_thm":bool
  out "file_extension_tgz":bool
  out "file_extension_swf":bool
  out "file_extension_ss":bool
  out "file_extension_sitx":bool
  out "file_extension_sit":bool
  out "file_extension_ses":bool
  out "file_extension_sea":bool
  out "file_extension_rtf":bool
  out "file_extension_rmvb":bool
  out "file_extension_rm":bool
  out "file_extension_rar":bool
  out "file_extension_ram":bool
  out "file_extension_qxd":bool
  out "file_extension_qbw":bool
  out "file_extension_qbb":bool
  out "file_extension_pub":bool
  out "file_extension_ptb":bool
  out "file_extension_pst":bool
  out "file_extension_psd":bool
  out "file_extension_ps":bool
  out "file_extension_pps":bool
  out "file_extension_png":bool
  out "file_extension_pdf":bool
  out "file_extension_ogg":bool
  out "file_extension_mswmm":bool
  out "file_extension_msi":bool
  out "file_extension_mpg":bool
  out "file_extension_mpeg":bool
  out "file_extension_mp4":bool
  out "file_extension_mp2":bool
  out "file_extension_mov":bool
  out "file_extension_mid":bool
  out "file_extension_mdb":bool
  out "file_extension_mcd":bool
  out "file_extension_m4v":bool
  out "file_extension_m4p":bool
  out "file_extension_m4b":bool
  out "file_extension_m4a":bool
  out "file_extension_log":bool
  out "file_extension_lnk":bool
  out "file_extension_jpg":bool
  out "file_extension_jpeg":bool
  out "file_extension_jar":bool
  out "file_extension_iso":bool
  out "file_extension_indd":bool
  out "file_extension_ifo":bool
  out "file_extension_html":bool
  out "file_extension_htm":bool
  out "file_extension_hqx":bool
  out "file_extension_gz":bool
  out "file_extension_gif":bool
  out "file_extension_flv":bool
  out "file_extension_fla":bool
  out "file_extension_exe":bool
  out "file_extension_eps":bool
  out "file_extension_eml":bool
  out "file_extension_dwg":bool
  out "file_extension_dvf":bool
  out "file_extension_dss":bool
  out "file_extension_doc":bool
  out "file_extension_dmg":bool
  out "file_extension_dll":bool
  out "file_extension_divx":bool
  out "file_extension_dat":bool
  out "file_extension_chm":bool
  out "file_extension_cdr":bool
  out "file_extension_cdl":bool
  out "file_extension_cda":bool
  out "file_extension_cbr":bool
  out "file_extension_cab":bool
  out "file_extension_bup":bool
  out "file_extension_bmp":bool
  out "file_extension_bin":bool
  out "file_extension_bat":bool
  out "file_extension_asx":bool
  out "file_extension_asf":bool
  out "file_extension_amr":bool
  out "file_extension_aiff":bool
  out "file_extension_aif":bool
  out "file_extension_ai":bool
  out "file_extension_ace":bool
  out "file_extension_7z":bool
  out "file_extension_3gp":bool
  out "female":bool
  out "feed_magnify":bool
  out "feed_key":bool
  out "feed_go":bool
  out "feed_error":bool
  out "feed_edit":bool
  out "feed_disk":bool
  out "feed_delete":bool
  out "feed_add":bool
  out "feed":bool
  out "fedora":bool
  out "fax":bool
  out "fatcow":bool
  out "factory":bool
  out "facebook":bool
  out "faberge_egg":bool
  out "eye_red":bool
  out "eye_close":bool
  out "eye":bool
  out "extract_foreground_objects":bool
  out "external":bool
  out "export_excel":bool
  out "exclamation":bool
  out "evernote":bool
  out "events":bool
  out "evacuator":bool
  out "escimo_pie":bool
  out "error_go":bool
  out "error_delete":bool
  out "error_add":bool
  out "error":bool
  out "envelope_string":bool
  out "envelope":bool
  out "entity":bool
  out "emotion_zedz":bool
  out "emotion_wink":bool
  out "emotion_whist":bool
  out "emotion_what":bool
  out "emotion_waii":bool
  out "emotion_waaaht":bool
  out "emotion_vampire":bool
  out "emotion_unshaven":bool
  out "emotion_unhappy":bool
  out "emotion_too_sad":bool
  out "emotion_tongue":bool
  out "emotion_tire":bool
  out "emotion_terminator":bool
  out "emotion_sweat":bool
  out "emotion_surrender":bool
  out "emotion_sure":bool
  out "emotion_suprised":bool
  out "emotion_stupid":bool
  out "emotion_star":bool
  out "emotion_spy":bool
  out "emotion_spiderman":bool
  out "emotion_smile":bool
  out "emotion_sleep":bool
  out "emotion_skull":bool
  out "emotion_silent":bool
  out "emotion_sick":bool
  out "emotion_shocked":bool
  out "emotion_shame":bool
  out "emotion_sad":bool
  out "emotion_red":bool
  out "emotion_rap":bool
  out "emotion_question":bool
  out "emotion_pumpkin":bool
  out "emotion_pirate":bool
  out "emotion_nosebleed":bool
  out "emotion_ninja":bool
  out "emotion_nerd":bool
  out "emotion_mummy":bool
  out "emotion_money":bool
  out "emotion_misdoubt":bool
  out "emotion_medic":bool
  out "emotion_matrix":bool
  out "emotion_mad":bool
  out "emotion_love":bool
  out "emotion_kissed":bool
  out "emotion_kiss":bool
  out "emotion_jason":bool
  out "emotion_japan":bool
  out "emotion_hypnotized":bool
  out "emotion_hungry":bool
  out "emotion_horror":bool
  out "emotion_hitler":bool
  out "emotion_happy":bool
  out "emotion_hand_flower":bool
  out "emotion_haha":bool
  out "emotion_grin":bool
  out "emotion_greedy":bool
  out "emotion_go":bool
  out "emotion_girl":bool
  out "emotion_ghost":bool
  out "emotion_gear":bool
  out "emotion_franken":bool
  out "emotion_flower_dead":bool
  out "emotion_fan":bool
  out "emotion_face_panda":bool
  out "emotion_face_monkey":bool
  out "emotion_eyes_droped":bool
  out "emotion_exciting":bool
  out "emotion_evolution":bool
  out "emotion_evilgrin":bool
  out "emotion_dribble":bool
  out "emotion_doubt":bool
  out "emotion_diver":bool
  out "emotion_devil":bool
  out "emotion_dead":bool
  out "emotion_david_blaine":bool
  out "emotion_darth_wader":bool
  out "emotion_cyclops":bool
  out "emotion_cry":bool
  out "emotion_crazy_rabbit":bool
  out "emotion_crazy":bool
  out "emotion_cool":bool
  out "emotion_confuse":bool
  out "emotion_confident":bool
  out "emotion_cold":bool
  out "emotion_clown":bool
  out "emotion_bye_bye":bool
  out "emotion_bubblegum":bool
  out "emotion_bloody":bool
  out "emotion_bigsmile":bool
  out "emotion_beaten":bool
  out "emotion_beat_brick":bool
  out "emotion_batman":bool
  out "emotion_baffle":bool
  out "emotion_bad_smelly":bool
  out "emotion_bad_egg":bool
  out "emotion_baby":bool
  out "emotion_angry":bool
  out "emotion_anger":bool
  out "emotion_angel":bool
  out "emotion_amazing":bool
  out "emotion_alien":bool
  out "emotion_ah":bool
  out "emotion_after_boom":bool
  out "emotion_adore":bool
  out "ember":bool
  out "emails_stack":bool
  out "emails":bool
  out "email_to_friend":bool
  out "email_send_receive":bool
  out "email_open_image":bool
  out "email_open":bool
  out "email_link":bool
  out "email_go":bool
  out "email_forward":bool
  out "email_error":bool
  out "email_edit":bool
  out "email_delete":bool
  out "email_attach":bool
  out "email_at_sign":bool
  out "email_air":bool
  out "email_add":bool
  out "email":bool
  out "elements":bool
  out "electric_guitar":bool
  out "ehow":bool
  out "egyptian_pyramid":bool
  out "education":bool
  out "edit_path":bool
  out "edit_mathematics":bool
  out "edit_free":bool
  out "edit_diff":bool
  out "edit_chain":bool
  out "echeck":bool
  out "ebay":bool
  out "earth_night":bool
  out "ear_listen":bool
  out "e_book_reader_white":bool
  out "e_book_reader_black":bool
  out "dynamite":bool
  out "dvd_link":bool
  out "dvd_key":bool
  out "dvd_go":bool
  out "dvd_error":bool
  out "dvd_edit":bool
  out "dvd_delete":bool
  out "dvd_add":bool
  out "dvd":bool
  out "drum":bool
  out "drugs_com":bool
  out "drop":bool
  out "drive_web":bool
  out "drive_user":bool
  out "drive_rename":bool
  out "drive_network":bool
  out "drive_magnify":bool
  out "drive_link":bool
  out "drive_key":bool
  out "drive_go":bool
  out "drive_error":bool
  out "drive_edit":bool
  out "drive_disk":bool
  out "drive_delete":bool
  out "drive_cd_empty":bool
  out "drive_cd":bool
  out "drive_burn":bool
  out "drive_add":bool
  out "drive":bool
  out "drink_empty":bool
  out "drink":bool
  out "drill":bool
  out "dribbble":bool
  out "drawer_open":bool
  out "drawer":bool
  out "draw_wave":bool
  out "draw_vertex":bool
  out "draw_star":bool
  out "draw_spiral":bool
  out "draw_smudge":bool
  out "draw_ring":bool
  out "draw_polyline":bool
  out "draw_polygon_curves":bool
  out "draw_polygon":bool
  out "draw_points":bool
  out "draw_path":bool
  out "draw_line":bool
  out "draw_island":bool
  out "draw_ink":bool
  out "draw_eraser":bool
  out "draw_ellipse":bool
  out "draw_dodge_burn":bool
  out "draw_convolve":bool
  out "draw_clone":bool
  out "draw_calligraphic":bool
  out "draw_airbrush":bool
  out "download_for_windows":bool
  out "download_for_mac":bool
  out "download_for_linux":bool
  out "download_cloud":bool
  out "download":bool
  out "down_jacket":bool
  out "dopplr":bool
  out "door_out":bool
  out "door_open":bool
  out "door_in":bool
  out "door":bool
  out "donut":bool
  out "domain_template":bool
  out "domain_names_advanced":bool
  out "domain_name_monetization":bool
  out "domain_name_investment":bool
  out "domain_legal_issues":bool
  out "domain_controversies":bool
  out "domain_buying_selling":bool
  out "dog":bool
  out "documents_email":bool
  out "document_yellow":bool
  out "document_white_torn":bool
  out "document_view_book":bool
  out "document_vertical":bool
  out "document_valid":bool
  out "document_tree":bool
  out "document_torn":bool
  out "document_todo":bool
  out "document_tag":bool
  out "document_stand":bool
  out "document_split":bool
  out "document_spacing":bool
  out "document_signature":bool
  out "document_shred":bool
  out "document_shapes":bool
  out "document_rename":bool
  out "document_redirect":bool
  out "document_red":bool
  out "document_quote":bool
  out "document_properties":bool
  out "document_prepare":bool
  out "document_plus":bool
  out "document_page_previous":bool
  out "document_page_next":bool
  out "document_page_last":bool
  out "document_page":bool
  out "document_num":bool
  out "document_notes":bool
  out "document_next":bool
  out "document_move":bool
  out "document_mark_as_final":bool
  out "document_margins":bool
  out "document_layout":bool
  out "document_inspector":bool
  out "document_inspect":bool
  out "document_insert":bool
  out "document_info":bool
  out "document_index":bool
  out "document_import":bool
  out "document_image_ver":bool
  out "document_image_hor":bool
  out "document_image":bool
  out "document_green":bool
  out "document_font_wizard":bool
  out "document_font":bool
  out "document_export":bool
  out "document_empty":bool
  out "document_editing":bool
  out "document_copies":bool
  out "document_comments":bool
  out "document_comment_below":bool
  out "document_comment_behind":bool
  out "document_comment_above":bool
  out "document_check_compatibility":bool
  out "document_center":bool
  out "document_break":bool
  out "document_black":bool
  out "document_background":bool
  out "document_back":bool
  out "do_not_disturb":bool
  out "dns_setting":bool
  out "dns":bool
  out "distribution_partnerships":bool
  out "disk_multiple":bool
  out "disk":bool
  out "dish":bool
  out "discover":bool
  out "disconnect":bool
  out "directory_listing":bool
  out "direction":bool
  out "dinersclub":bool
  out "digital_signature_pen":bool
  out "digital_signature":bool
  out "digg":bool
  out "dice":bool
  out "diamond":bool
  out "dialog":bool
  out "diagramm":bool
  out "diagnostic_chart":bool
  out "devianart":bool
  out "desktop":bool
  out "designmoo":bool
  out "design_float":bool
  out "derivatives":bool
  out "delicious":bool
  out "delete":bool
  out "decimal_more":bool
  out "decimal_less":bool
  out "debian":bool
  out "ddr_memory":bool
  out "date_task":bool
  out "date_relation":bool
  out "date_previous_gray":bool
  out "date_previous":bool
  out "date_next_gray":bool
  out "date_next":bool
  out "date_magnify":bool
  out "date_link":bool
  out "date_go":bool
  out "date_error":bool
  out "date_edit":bool
  out "date_delete":bool
  out "date_add":bool
  out "date":bool
  out "database_yellow":bool
  out "database_table":bool
  out "database_server":bool
  out "database_save":bool
  out "database_refresh":bool
  out "database_red":bool
  out "database_link":bool
  out "database_lightning":bool
  out "database_key":bool
  out "database_green":bool
  out "database_go":bool
  out "database_gear":bool
  out "database_error":bool
  out "database_edit":bool
  out "database_delete":bool
  out "database_connect":bool
  out "database_blue":bool
  out "database_black":bool
  out "database_add":bool
  out "database":bool
  out "data_table":bool
  out "data_sort":bool
  out "data_grid":bool
  out "data_field":bool
  out "data_chooser":bool
  out "dashboard":bool
  out "cutter":bool
  out "cutlery":bool
  out "cutleries":bool
  out "cut_red":bool
  out "cut":bool
  out "cushion":bool
  out "curtain":bool
  out "cursor":bool
  out "curriculum_vitae":bool
  out "cup_silver":bool
  out "cup_link":bool
  out "cup_key":bool
  out "cup_gold":bool
  out "cup_go":bool
  out "cup_error":bool
  out "cup_edit":bool
  out "cup_delete":bool
  out "cup_bronze":bool
  out "cup_add":bool
  out "cup":bool
  out "css_valid":bool
  out "css_go":bool
  out "css_delete":bool
  out "css_add":bool
  out "css_3":bool
  out "css":bool
  out "cruise_ship":bool
  out "crown_silver":bool
  out "crown_gold":bool
  out "crown_bronze":bool
  out "cross_shield":bool
  out "cross_promotion_selling":bool
  out "cross":bool
  out "cricket":bool
  out "creditcards":bool
  out "credit":bool
  out "creative_commons":bool
  out "counter":bool
  out "copyleft":bool
  out "copying_and_distribution":bool
  out "cooler":bool
  out "cookies":bool
  out "cookie_chocolate":bool
  out "convert_gray_to_color":bool
  out "convert_color_to_gray":bool
  out "conversion_of_currency":bool
  out "controller_error":bool
  out "controller_delete":bool
  out "controller_add":bool
  out "controller":bool
  out "controlbar":bool
  out "control_stop_blue":bool
  out "control_stop":bool
  out "control_start_blue":bool
  out "control_start":bool
  out "control_rewind_blue":bool
  out "control_rewind":bool
  out "control_repeat_blue":bool
  out "control_repeat":bool
  out "control_power_blue":bool
  out "control_power":bool
  out "control_play_blue":bool
  out "control_play":bool
  out "control_pause_record":bool
  out "control_pause_blue":bool
  out "control_pause":bool
  out "control_panel_branding":bool
  out "control_panel_access":bool
  out "control_panel":bool
  out "control_fastforward_blue":bool
  out "control_fastforward":bool
  out "control_equalizer_blue":bool
  out "control_equalizer":bool
  out "control_end_blue":bool
  out "control_end":bool
  out "control_eject_blue":bool
  out "control_eject":bool
  out "control_cursor_blue":bool
  out "control_cursor":bool
  out "contrast_low":bool
  out "contrast_increase":bool
  out "contrast_high":bool
  out "contrast_decrease":bool
  out "contrast":bool
  out "contact_email":bool
  out "construction":bool
  out "connect":bool
  out "computer_link":bool
  out "computer_key":bool
  out "computer_go":bool
  out "computer_error":bool
  out "computer_edit":bool
  out "computer_delete":bool
  out "computer_add":bool
  out "computer":bool
  out "compress":bool
  out "compile_warning":bool
  out "compile_error":bool
  out "compile":bool
  out "compass":bool
  out "company_generosity":bool
  out "comments_twitter":bool
  out "comments_facebook":bool
  out "comments_delete":bool
  out "comments_add":bool
  out "comments":bool
  out "comment_white":bool
  out "comment_twitter_retwit":bool
  out "comment_twitter_box":bool
  out "comment_twitter":bool
  out "comment_google":bool
  out "comment_facebook_box":bool
  out "comment_facebook":bool
  out "comment_edit":bool
  out "comment_delete":bool
  out "comment_box":bool
  out "comment_add":bool
  out "comment":bool
  out "combo_box":bool
  out "columnchart":bool
  out "column_two":bool
  out "column_tree":bool
  out "column_single":bool
  out "column_right":bool
  out "column_one":bool
  out "column_left":bool
  out "column_four":bool
  out "column_double":bool
  out "color_wheel":bool
  out "color_swatches":bool
  out "color_swatch":bool
  out "color_picker_alternative":bool
  out "color_picker":bool
  out "color_management":bool
  out "color_gradient":bool
  out "color_adjustment_red":bool
  out "color_adjustment_green":bool
  out "color_adjustment_blue":bool
  out "color_adjustment":bool
  out "cold":bool
  out "coins_in_hand":bool
  out "coins_delete":bool
  out "coins_add":bool
  out "coins":bool
  out "coin_stack_gold":bool
  out "coin_single_silver":bool
  out "coin_single_gold":bool
  out "coin_single_cooper":bool
  out "cog_go":bool
  out "cog_error":bool
  out "cog_edit":bool
  out "cog_delete":bool
  out "cog_add":bool
  out "cog":bool
  out "code":bool
  out "cocacola":bool
  out "co2":bool
  out "clown_fish":bool
  out "clock_stop":bool
  out "clock_select_remain":bool
  out "clock_red":bool
  out "clock_play":bool
  out "clock_pause":bool
  out "clock_moon_phase":bool
  out "clock_link":bool
  out "clock_history_frame":bool
  out "clock_go":bool
  out "clock_error":bool
  out "clock_edit":bool
  out "clock_delete":bool
  out "clock_add":bool
  out "clock_45":bool
  out "clock_15":bool
  out "clock":bool
  out "clipboard_sign_out":bool
  out "clipboard_sign":bool
  out "clipboard_invoice":bool
  out "clipboard_empty":bool
  out "clip_splitter":bool
  out "client_account_template":bool
  out "cirrus":bool
  out "circus":bool
  out "cinema_ticket":bool
  out "cigarette":bool
  out "church":bool
  out "christmas_tree":bool
  out "chocolate_bite":bool
  out "chocolate":bool
  out "chinese_noodles":bool
  out "children_cap":bool
  out "chiken_leg":bool
  out "chess_tower":bool
  out "chess_horse":bool
  out "cheque":bool
  out "chefs_hat":bool
  out "cheese":bool
  out "checkerboard":bool
  out "check_box":bool
  out "chartplotter":bool
  out "chart_up_color":bool
  out "chart_stock":bool
  out "chart_pie_link":bool
  out "chart_pie_error":bool
  out "chart_pie_edit":bool
  out "chart_pie_delete":bool
  out "chart_pie_alternative":bool
  out "chart_pie_add":bool
  out "chart_pie":bool
  out "chart_organisation_delete":bool
  out "chart_organisation_add":bool
  out "chart_organisation":bool
  out "chart_line_link":bool
  out "chart_line_error":bool
  out "chart_line_edit":bool
  out "chart_line_delete":bool
  out "chart_line_add":bool
  out "chart_line":bool
  out "chart_down_color":bool
  out "chart_curve_link":bool
  out "chart_curve_go":bool
  out "chart_curve_error":bool
  out "chart_curve_edit":bool
  out "chart_curve_delete":bool
  out "chart_curve_add":bool
  out "chart_curve":bool
  out "chart_column_2":bool
  out "chart_column":bool
  out "chart_bullseye":bool
  out "chart_bar_link":bool
  out "chart_bar_error":bool
  out "chart_bar_edit":bool
  out "chart_bar_delete":bool
  out "chart_bar_add":bool
  out "chart_bar":bool
  out "change_password":bool
  out "chameleon":bool
  out "chair":bool
  out "ceo":bool
  out "centroid":bool
  out "centos":bool
  out "celsius":bool
  out "cd_go":bool
  out "cd_eject":bool
  out "cd_edit":bool
  out "cd_delete":bool
  out "cd_case_empty":bool
  out "cd_case":bool
  out "cd_burn":bool
  out "cd_add":bool
  out "cd":bool
  out "cctv_camera":bool
  out "caution_radiation":bool
  out "caution_high_voltage":bool
  out "caution_board":bool
  out "caution_biohazard":bool
  out "cats_display":bool
  out "caterpillar":bool
  out "category_item_select":bool
  out "category_item":bool
  out "category_group_select":bool
  out "category_group":bool
  out "category":bool
  out "categories":bool
  out "cat":bool
  out "cash_terminal":bool
  out "cash_stack":bool
  out "cash_register_2":bool
  out "cash_register":bool
  out "cart_remove":bool
  out "cart_put":bool
  out "cart_go":bool
  out "cart_full":bool
  out "cart_error":bool
  out "cart_edit":bool
  out "cart_delete":bool
  out "cart_add":bool
  out "cart":bool
  out "cargo":bool
  out "cards_binds":bool
  out "cards_bind_address":bool
  out "cards":bool
  out "card_solo":bool
  out "card_save":bool
  out "card_sapphire":bool
  out "card_money":bool
  out "card_miles":bool
  out "card_ipod":bool
  out "card_import":bool
  out "card_gold":bool
  out "card_gift_2":bool
  out "card_gift":bool
  out "card_front":bool
  out "card_export":bool
  out "card_echeck":bool
  out "card_discover_novus":bool
  out "card_discover_black":bool
  out "card_debit":bool
  out "card_credit":bool
  out "card_chip_silver":bool
  out "card_chip_gold":bool
  out "card_chase":bool
  out "card_bank":bool
  out "card_back":bool
  out "card_apple":bool
  out "card_amex_green":bool
  out "card_amex_gray":bool
  out "card_amex_gold":bool
  out "card_amazon":bool
  out "car_taxi":bool
  out "car_delete":bool
  out "car_add":bool
  out "car":bool
  out "cap":bool
  out "canvas_size":bool
  out "canvas":bool
  out "candy_cane":bool
  out "candlestickchart":bool
  out "candle_2":bool
  out "candle":bool
  out "cancel":bool
  out "camera_small":bool
  out "camera_link":bool
  out "camera_lens":bool
  out "camera_go":bool
  out "camera_error":bool
  out "camera_edit":bool
  out "camera_delete":bool
  out "camera_black":bool
  out "camera_add":bool
  out "camera":bool
  out "camcorder":bool
  out "calendar_view_week":bool
  out "calendar_view_month":bool
  out "calendar_view_day":bool
  out "calendar_link":bool
  out "calendar_edit":bool
  out "calendar_delete":bool
  out "calendar_copy":bool
  out "calendar_add":bool
  out "calendar":bool
  out "calculator_link":bool
  out "calculator_error":bool
  out "calculator_edit":bool
  out "calculator_delete":bool
  out "calculator_black":bool
  out "calculator_add":bool
  out "calculator":bool
  out "cake":bool
  out "cactus":bool
  out "buzz":bool
  out "buttonbar":bool
  out "button":bool
  out "butterfly":bool
  out "bus":bool
  out "burro":bool
  out "bullet_yellow":bool
  out "bullet_wrench":bool
  out "bullet_world":bool
  out "bullet_word":bool
  out "bullet_white":bool
  out "bullet_vector":bool
  out "bullet_valid":bool
  out "bullet_user":bool
  out "bullet_up":bool
  out "bullet_toggle_plus":bool
  out "bullet_toggle_minus":bool
  out "bullet_textfield":bool
  out "bullet_table":bool
  out "bullet_star":bool
  out "bullet_red":bool
  out "bullet_purple":bool
  out "bullet_powerpoint":bool
  out "bullet_pink":bool
  out "bullet_picture":bool
  out "bullet_php":bool
  out "bullet_palette":bool
  out "bullet_orange":bool
  out "bullet_office":bool
  out "bullet_medal":bool
  out "bullet_magnify":bool
  out "bullet_link":bool
  out "bullet_lightning":bool
  out "bullet_key":bool
  out "bullet_green":bool
  out "bullet_go":bool
  out "bullet_gear":bool
  out "bullet_flash":bool
  out "bullet_find":bool
  out "bullet_feed":bool
  out "bullet_excel":bool
  out "bullet_error":bool
  out "bullet_edit":bool
  out "bullet_dvd":bool
  out "bullet_down":bool
  out "bullet_document":bool
  out "bullet_disk":bool
  out "bullet_delete":bool
  out "bullet_database":bool
  out "bullet_connect":bool
  out "bullet_code_red":bool
  out "bullet_code":bool
  out "bullet_chart":bool
  out "bullet_cd":bool
  out "bullet_camera":bool
  out "bullet_burn":bool
  out "bullet_bulb_on":bool
  out "bullet_bulb_off":bool
  out "bullet_bug":bool
  out "bullet_brush":bool
  out "bullet_blue":bool
  out "bullet_black":bool
  out "bullet_bell":bool
  out "bullet_back":bool
  out "bullet_attach":bool
  out "bullet_arrow_up":bool
  out "bullet_arrow_top":bool
  out "bullet_arrow_right_2":bool
  out "bullet_arrow_right":bool
  out "bullet_arrow_left_2":bool
  out "bullet_arrow_left":bool
  out "bullet_arrow_down":bool
  out "bullet_arrow_bottom":bool
  out "bullet_archive":bool
  out "bullet_add":bool
  out "bulb":bool
  out "building_link":bool
  out "building_key":bool
  out "building_go":bool
  out "building_error":bool
  out "building_edit":bool
  out "building_delete":bool
  out "building_add":bool
  out "building":bool
  out "bug_link":bool
  out "bug_go":bool
  out "bug_error":bool
  out "bug_edit":bool
  out "bug_delete":bool
  out "bug_add":bool
  out "bug":bool
  out "bucket_truck":bool
  out "bubblechart":bool
  out "brushes":bool
  out "broom":bool
  out "brightkite":bool
  out "briefcase":bool
  out "bricks":bool
  out "brick_link":bool
  out "brick_go":bool
  out "brick_error":bool
  out "brick_edit":bool
  out "brick_delete":bool
  out "brick_add":bool
  out "brick":bool
  out "breeze":bool
  out "bread":bool
  out "brain_trainer":bool
  out "brain":bool
  out "boxing_glove":bool
  out "box_search":bool
  out "box_open":bool
  out "box_front":bool
  out "box_down":bool
  out "box_closed":bool
  out "box":bool
  out "bow":bool
  out "border_color":bool
  out "border_2_top":bool
  out "border_2_right":bool
  out "border_2_outer":bool
  out "border_2_left":bool
  out "border_2_bottom":bool
  out "border_1d_top":bool
  out "border_1d_right":bool
  out "border_1d_left":bool
  out "border_1d_bottom":bool
  out "border_1d_around":bool
  out "border_1_ver":bool
  out "border_1_top":bool
  out "border_1_right":bool
  out "border_1_outer":bool
  out "border_1_none":bool
  out "border_1_middle":bool
  out "border_1_left":bool
  out "border_1_hor":bool
  out "border_1_bottom":bool
  out "border_1":bool
  out "boomerang":bool
  out "bookshelf":bool
  out "books_stack":bool
  out "books":bool
  out "bookmark_red":bool
  out "bookmark":bool
  out "book_spelling":bool
  out "book_previous":bool
  out "book_picture":bool
  out "book_open":bool
  out "book_next":bool
  out "book_link":bool
  out "book_key":bool
  out "book_keeping":bool
  out "book_go":bool
  out "book_error":bool
  out "book_edit":bool
  out "book_delete":bool
  out "book_addresses":bool
  out "book_add":bool
  out "book":bool
  out "bomb":bool
  out "board_game":bool
  out "bluetooth":bool
  out "blueprints":bool
  out "blueprint_horizontal":bool
  out "blueprint":bool
  out "blogs":bool
  out "blogger":bool
  out "blackboard_sum":bool
  out "blackboard_steps":bool
  out "blackboard_empty":bool
  out "blackboard_drawing":bool
  out "blackberry_white":bool
  out "blackberry_messenger":bool
  out "blackberry":bool
  out "bios":bool
  out "bin_recycle":bool
  out "bin_empty":bool
  out "bin_closed":bool
  out "bin":bool
  out "billiard_marker":bool
  out "bell_link":bool
  out "bell_go":bool
  out "bell_error":bool
  out "bell_delete":bool
  out "bell_add":bool
  out "bell":bool
  out "beer":bool
  out "bedo":bool
  out "bed":bool
  out "bean":bool
  out "beaker_empty":bool
  out "beaker":bool
  out "battery_plug":bool
  out "battery_low":bool
  out "battery_half":bool
  out "battery_full":bool
  out "battery_charge":bool
  out "battery":bool
  out "baton":bool
  out "basket_remove":bool
  out "basket_put":bool
  out "basket_go":bool
  out "basket_full":bool
  out "basket_error":bool
  out "basket_edit":bool
  out "basket_delete":bool
  out "basket_add":bool
  out "basket":bool
  out "barcode_2d":bool
  out "barcode":bool
  out "barchart":bool
  out "bank":bool
  out "bandaid":bool
  out "bamboos":bool
  out "bamboo":bool
  out "baloon_2_empty":bool
  out "baloon_2":bool
  out "baloon":bool
  out "ballon":bool
  out "balance_unbalance":bool
  out "balance":bool
  out "baggage_cart_box":bool
  out "baggage_cart":bool
  out "backup_manager":bool
  out "backpack":bool
  out "baby_bottle":bool
  out "ax":bool
  out "award_star_silver_3":bool
  out "award_star_silver_2":bool
  out "award_star_silver_1":bool
  out "award_star_gold_3":bool
  out "award_star_gold_2":bool
  out "award_star_gold_1":bool
  out "award_star_delete":bool
  out "award_star_bronze_3":bool
  out "award_star_bronze_2":bool
  out "award_star_bronze_1":bool
  out "award_star_add":bool
  out "autos":bool
  out "auction_hammer_gavel":bool
  out "attribution":bool
  out "attributes_display":bool
  out "attach":bool
  out "atm":bool
  out "at_sign":bool
  out "asterisk_yellow":bool
  out "asterisk_orange":bool
  out "ask_and_answer":bool
  out "artwork":bool
  out "arrow_up":bool
  out "arrow_undo":bool
  out "arrow_turn_right":bool
  out "arrow_turn_left":bool
  out "arrow_switch":bool
  out "arrow_rotate_clockwise":bool
  out "arrow_rotate_anticlockwise":bool
  out "arrow_right":bool
  out "arrow_refresh_small":bool
  out "arrow_refresh":bool
  out "arrow_redo":bool
  out "arrow_out":bool
  out "arrow_merge":bool
  out "arrow_left":bool
  out "arrow_join":bool
  out "arrow_inout":bool
  out "arrow_in":bool
  out "arrow_down":bool
  out "arrow_divide":bool
  out "arrow_branch":bool
  out "areachart":bool
  out "arch_linux":bool
  out "application_xp_terminal":bool
  out "application_xp":bool
  out "application_view_tile":bool
  out "application_view_list":bool
  out "application_view_icons":bool
  out "application_view_gallery":bool
  out "application_view_detail":bool
  out "application_view_columns":bool
  out "application_tile_vertical":bool
  out "application_tile_horizontal":bool
  out "application_split":bool
  out "application_side_tree":bool
  out "application_side_list":bool
  out "application_side_expand":bool
  out "application_side_contract":bool
  out "application_side_boxes":bool
  out "application_put":bool
  out "application_osx_terminal":bool
  out "application_osx":bool
  out "application_link":bool
  out "application_lightning":bool
  out "application_key":bool
  out "application_home":bool
  out "application_go":bool
  out "application_get":bool
  out "application_from_storage":bool
  out "application_form_magnify":bool
  out "application_form_edit":bool
  out "application_form_delete":bool
  out "application_form_add":bool
  out "application_form":bool
  out "application_error":bool
  out "application_edit":bool
  out "application_double":bool
  out "application_delete":bool
  out "application_control_bar":bool
  out "application_cascade":bool
  out "application_add":bool
  out "application":bool
  out "apple_half":bool
  out "apple_corp":bool
  out "apple":bool
  out "aol_messenger":bool
  out "aol_mail":bool
  out "anti_xss":bool
  out "angel":bool
  out "android":bool
  out "anchor":bool
  out "american_express":bool
  out "all_right_reserved":bool
  out "alitalk":bool
  out "align_right":bool
  out "align_none":bool
  out "align_middle":bool
  out "align_left":bool
  out "align_compact":bool
  out "align_center":bool
  out "align_bellow":bool
  out "align_above":bool
  out "alarm_bell":bool
  out "aim_messenger":bool
  out "agp":bool
  out "advertising":bool
  out "advanced_data_grid":bool
  out "administrator":bool
  out "add":bool
  out "active_sessions":bool
  out "action_log":bool
  out "acoustic_guitar":bool
  out "acorn":bool
  out "account_balances":bool
  out "accordion":bool
  out "accept":bool
  out "64_bit":bool
  out "32_bit":bool
  out "3d_glasses":bool
  out "zootool":bool
  out "zoom_selection":bool
  out "zoom_refresh":bool
  out "zoom_out":bool
  out "zoom_layer":bool
  out "zoom_last":bool
  out "zoom_in":bool
  out "zoom_fit":bool
  out "zoom_extend":bool
  out "zoom_actual_equal":bool
  out "zoom_actual":bool
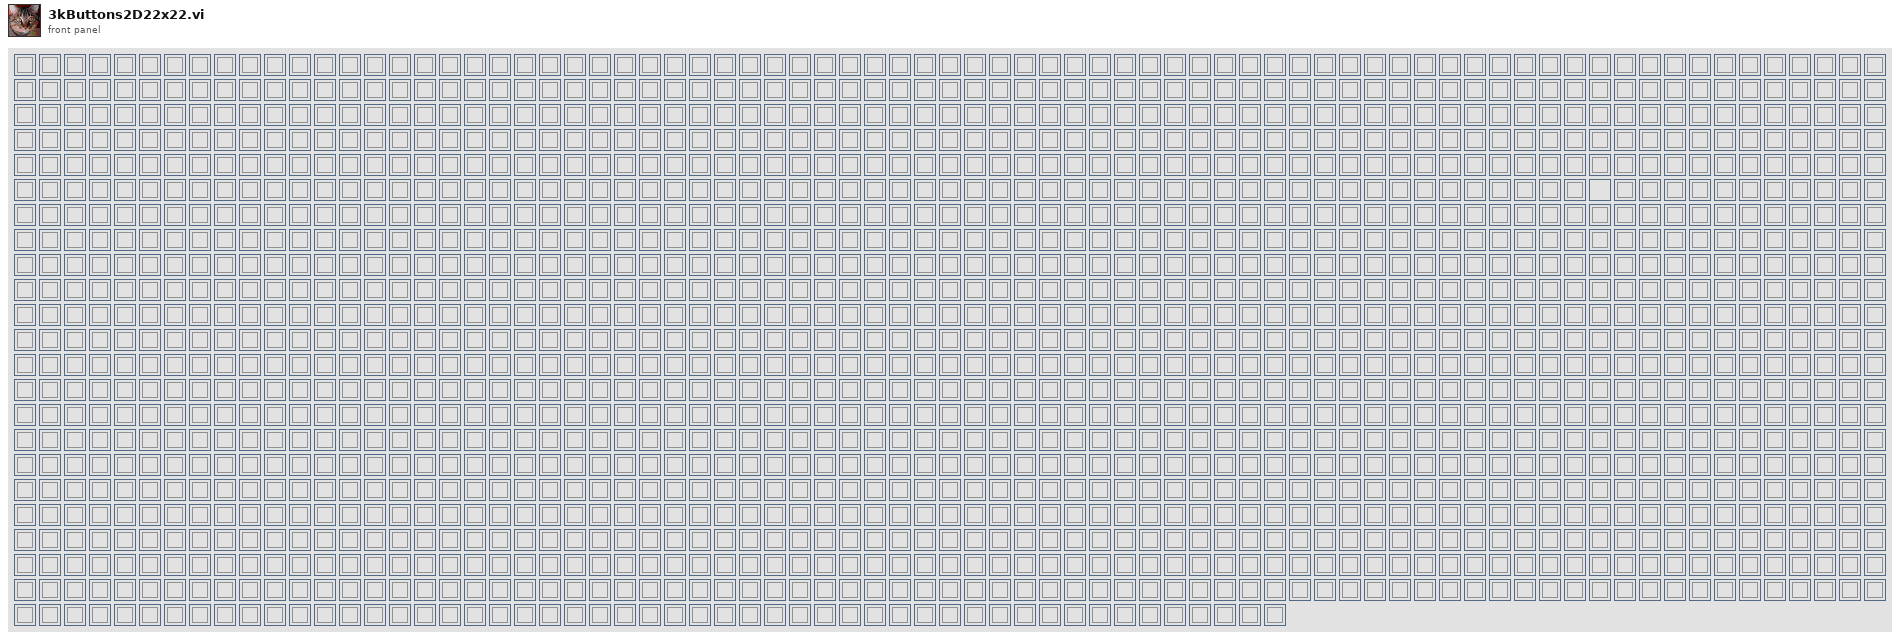
[diagram p1: front panel]
diagram:
